vi "@create.vi"(8 "error in (no error)":errorcluster, 11 "config":T1={"num letters"=0, "num guesses"=0, "default color"=15000804, "match color"=1689600, "half match color"=16766994, "no match color"=5263440, "dictonary"=[]}) -> (0 "error out":errorcluster, 3 "Worder out":refnum<class "Worder.lvclass">)   [LabVIEW 2020, in "Worder.lvclass"]
uses:
  Worder.lvclass
  config.ctl
  letter_box.ctl
  keyboard.ctl
  letter_box_small.ctl
  Worder.lvclass/Worder.ctl
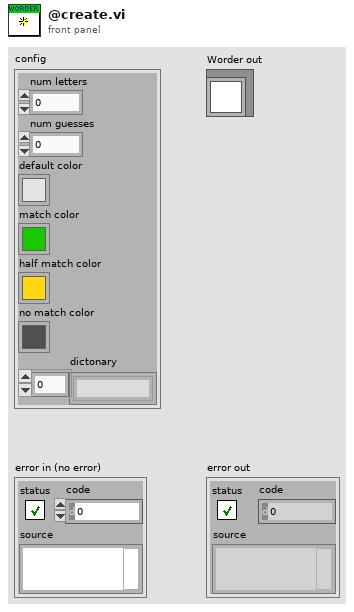
[diagram p1: front panel]
types:
  T1 = typedef "Worder.lvclass/config.ctl" = cluster{"num letters":i32, "num guesses":i32, "default color":u32, "match color":u32, "half match color":u32, "no match color":u32, "dictonary":string[]}
  T2 = typedef "Worder.lvclass/keyboard.ctl" = cluster{"A":T3, "B":T3, "C":T3, "D":T3, "E":T3, "F":T3, "G":T3, "H":T3, "I":T3, "J":T3, "K":T3, "L":T3, "M":T3, "N":T3, "O":T3, "P":T3, "Q":T3, "R":T3, "S":T3, "T":T3, "U":T3, "V":T3, "W":T3, "X":T3, "Y":T3, "Z":T3}
  T3 = typedef "Worder.lvclass/letter_box_small.ctl" = cluster{"color":u32, "char":string}
  T4 = typedef "Worder.lvclass/letter_box.ctl" = cluster{"color":u32, "char":string}
  T5 = cluster{"[0]":T3, "[1]":T3, "[2]":T3, "[3]":T3, "[4]":T3, "[5]":T3, "[6]":T3, "[7]":T3, "[8]":T3, "[9]":T3, "[10]":T3, "[11]":T3, "[12]":T3, "[13]":T3, "[14]":T3, "[15]":T3, "[16]":T3, "[17]":T3, "[18]":T3, "[19]":T3, "[20]":T3, "[21]":T3, "[22]":T3, "[23]":T3, "[24]":T3, "[25]":T3}
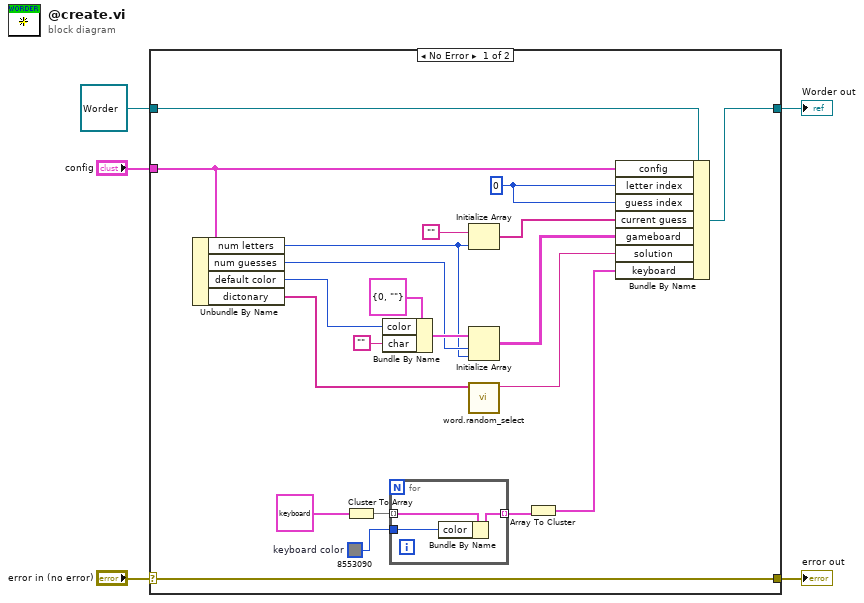
[diagram p0: block diagram]
diagram:
  n1 = case shown="No Error" "error in (no error)" {
    selector: "error in (no error)" -> [w26 w31]
    tunnel: [w26 w31] -> w4
    tunnel: [w21 w30] -> w2
    tunnel: refnum<class "Worder.lvclass"> refnum ("Worder in") -> [w22 w30]
    tunnel: "config" -> [w20 _]
    frame No Error {
      w6 = u32 8553090  # keyboard color
      w19 = 0 ("letter index")
      n2 = Unbundle By Name(w20) -> ("num letters"=w12:i32, "num guesses"=w13:i32, "default color"=w7:u32, "dictonary"=w14:string[])
      n3 = Cluster To Array(cluster=T2 {"A"={"color"=3815996, "char"="A"}, "B"={"color"=3815996, "char"="B"}, "C"={"color"=3815996, "char"="C"}, "D"={"color"=3815996, "char"="D"}, "E"={"color"=3815996, "char"="E"}, "F"={"color"=3815996, "char"="F"}, "G"={"color"=3815996, "char"="G"}, "H"={"color"=3815996, "char"="H"}, "I"={"color"=3815996, "char"="I"}, "J"={"color"=3815996, "char"="J"}, "K"={"color"=3815996, "char"="K"}, "L"={"color"=3815996, "char"="L"}, "M"={"color"=3815996, "char"="M"}, "N"={"color"=3815996, "char"="N"}, "O"={"color"=3815996, "char"="O"}, "P"={"color"=3815996, "char"="P"}, "Q"={"color"=3815996, "char"="Q"}, "R"={"color"=3815996, "char"="R"}, "S"={"color"=3815996, "char"="S"}, "T"={"color"=3815996, "char"="T"}, "U"={"color"=3815996, "char"="U"}, "V"={"color"=3815996, "char"="V"}, "W"={"color"=3815996, "char"="W"}, "X"={"color"=3815996, "char"="X"}, "Y"={"color"=3815996, "char"="Y"}, "Z"={"color"=3815996, "char"="Z"}} ("keyboard")) -> (array=w9:T3[])
      n4 = Bundle By Name(cluster=T4 {"color"=0, "char"=""} ("0"), "color"=w7, "char"="") -> (w24:T4)
      n5 = for {
        tunnel: w9 -> [w29] mode=indexing
        tunnel: [w28] -> w8 mode=indexing
        tunnel: w6 -> [w27]
        n6 = Bundle By Name(cluster=w29, "color"=w27) -> (w28:T3)
      }
      n7 = Initialize Array("", w12) -> (w17:string[])
      n8 = Initialize Array(w24, w13, w12) -> (w16:T4[][])
      n9 = call "word.random_select.vi"("dictonary"=w14) -> ("solution"=w15:string)  [unwired: 10 in]
      n10 = Array To Cluster(array=w8) -> (cluster=w10:T5)
      n11 = Bundle By Name(cluster=w22, "config"=w20, "letter index"=w19, "guess index"=w19, "current guess"=w17, "gameboard"=w16, "solution"=w15, "keyboard"=w10) -> (w21:refnum<class "Worder.lvclass">)
    }
    frame Error {
    }
  }
  "error out" <- w4
  "Worder out" <- w2
